vi "Receive Messages.vi"(8 "error in":errorcluster, 10 "Source":string, 11 "Worker in":refnum<class "Communicator Worker.lvclass">) -> (0 "error out":errorcluster, 2 "IMessages":refnum<class "IMessage.lvclass">[](array[class]), 3 "Worker out":refnum<class "Communicator Worker.lvclass">)   [LabVIEW 2024, in "Communicator Worker.lvlib" / "Communicator Worker.lvclass"]
uses:
  Communicator Worker.lvclass
  Interfaces/IMessage/IMessage.lvclass
  Communicator Worker.lvclass/Communicator Worker.ctl
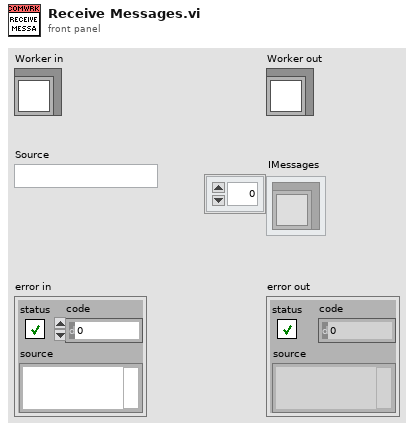
[diagram p1: front panel]
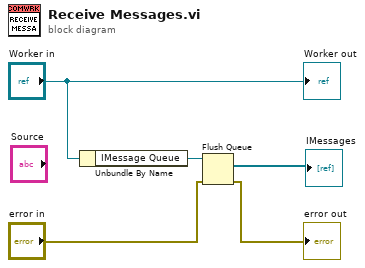
[diagram p0: block diagram]
diagram:
  n1 = Unbundle By Name("Worker in") -> ("IMessage Queue"=w4:refnum<queue>)
  n2 = Flush Queue(queue=w4, error in (no error)="error in") -> (remaining elements=→"IMessages":refnum<class "IMessage.lvclass">[], error out=→"error out":errorcluster)  [unwired: 1 out]
  "Worker out" <- "Worker in"
